vi "SetupDefault.vi"(8 "error in (no error)":errorcluster, 10 "Alias":string, 11 "NetA_RSZVL in":refnum<class "NetA_RSZVL.lvclass">) -> (0 "error out":errorcluster, 3 "NetA_RSZVL out":refnum<class "NetA_RSZVL.lvclass">)   [LabVIEW 2014, in "NetA_RSZVL.lvclass"]
uses:
  NetA_RSZVL.lvclass
  NetA_RSZVL.lvclass/NetA_RSZVL.ctl
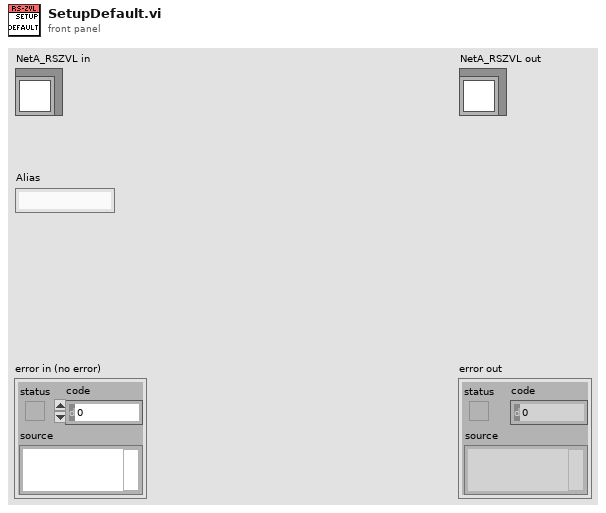
[diagram p1: front panel]
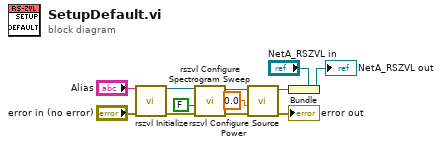
[diagram p0: block diagram]
diagram:
  n1 = call "rszvl Initialize.vi"("VISA resource name"="Alias", "error in (no error)"="error in (no error)") -> ("VISA resource name out"=w8:refnum<visa-resource-name>, "error out"=w7:errorcluster)  [unwired: 12 in]
  n2 = call "rszvl Configure Spectrogram Sweep.vi"("error in (no error)"=w7, "Continuous (On)"=FALSE, "VISA resource name"=w8) -> ("error out"=w4:errorcluster, "VISA resource name out"=w5:refnum<visa-resource-name>)  [unwired: 7 in]
  n3 = call "rszvl Configure Source Power.vi"("error in (no error)"=w4, "Source Power (-10.0)"=0.0, "VISA resource name"=w5) -> ("error out"=→"error out":errorcluster, "VISA resource name out"=w2:refnum<visa-resource-name>)  [unwired: 7 in]
  n4 = Bundle(cluster="NetA_RSZVL in", w2) -> (→"NetA_RSZVL out":refnum<class "NetA_RSZVL.lvclass">)
